vi "Pascal Matrix (DBL).vi"(11 "matrix size":i32) -> (0 "error":i32, 3 "Pascal Matrix":T1)   [LabVIEW 2018, in "NI_AALPro.lvlib"]
uses:
  NI_AALPro.lvlib
  RealMatrix.ctl
  NI_Matrix.lvlib
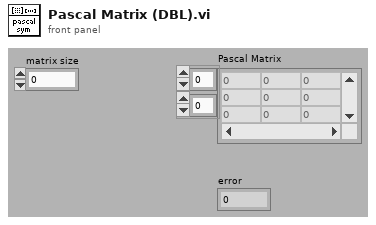
[diagram p1: front panel]
types:
  T1 = typedef "NI_Matrix.lvlib/RealMatrix.ctl" = dbl[][]
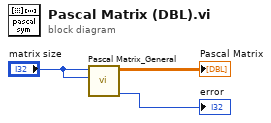
[diagram p0: block diagram]
diagram:
  n1 = call "Pascal Matrix_General.vi"("columns"="matrix size", "rows"="matrix size") -> ("error"=→"error":i32, "Pascal Matrix"=→"Pascal Matrix":dbl[][])  [unwired: 8 in]
